vi "Normalize Waveform.vi"(8 "error in (no error)":errorcluster, 11 "waveform in":waveform(dbl)) -> (0 "error out":errorcluster, 1 "offset":dbl format="%0.2f", 2 "scale":dbl format="%0.2f", 3 "normalized waveform":waveform(dbl))   [LabVIEW 2013]
doc: "Determines the <B>scale</B> and <B>offset</B> necessary to transform the waveform data so that its maximum is 1.00 and its minimum is -1.00."
uses:
  NI_AALBase.lvlib
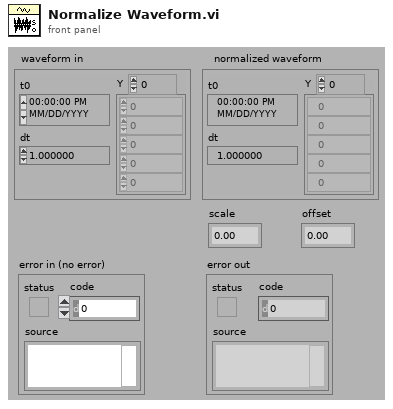
[diagram p1: front panel]
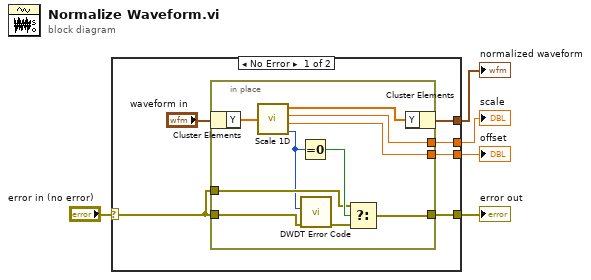
[diagram p0: block diagram]
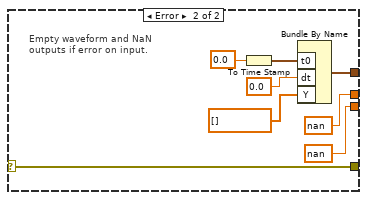
[diagram p2: hidden frame]
diagram:
  n1 = case shown="No Error" "error in (no error)" {
    selector: "error in (no error)" -> [w10 w29]
    tunnel: [w9 w26] -> w5
    tunnel: [w6 nan ("offset")] -> w4
    tunnel: [w7 nan ("scale")] -> w3
    tunnel: [w8 w29] -> w2
    frame No Error {
      n2 = in-place {
        in-place-border: w10 -> [w17]
        in-place-border: w10 -> [w16]
        in-place-border: [w14] -> w8
        in-place-border: [w13] -> w7
        in-place-border: [w12] -> w6
        n3 = in-place-cluster #1("waveform in") -> ("Y"=w21:dbl[])
        n4 = call "Scale 1D.vi"("X"=w21) -> ("Y=(X-offset)/scale"=w20:dbl[], "scale"=w13:dbl, "offset"=w12:dbl, "error"=w15:i32)
        n5 = Equal To 0?(x=w15) -> (x = 0?=w18:bool)
        n6 = call "DWDT Error Code.vi"("error in (no error)"=w17, "error code"=w15) -> ("error out"=w19:errorcluster)  [unwired: 9 out]
        n7 = Select(t=w16, s=w18, f=w19) -> (s? t:f=w14:errorcluster)
        n8 = in-place-cluster #1("Y"=w20) -> (w9:waveform(dbl))
      }
    }
    frame Error {
      # "Empty waveform and NaN\noutputs if error on input."
      n9 = To Time Stamp(1:0.0 ("t0")) -> (0:w22:timestamp)
      n10 = Bundle By Name("t0"=w22, "dt"=0.0, "Y"=dbl[] []) -> (w26:waveform(dbl))  [unwired: 1 out]
    }
  }
  "normalized waveform" <- w5
  "scale" <- w3
  "offset" <- w4
  "error out" <- w2
